vi "EAGLE Setup Screen V3.vi"(9 "TableIn":string[][](table)) -> (1 "TableOut":string[][](table), 2 "Exit":bool)   [LabVIEW 2015]
uses:
  Controls/Eagle Data.ctl
panel:
  in  "Down Button":bool
  in  "Up Button":bool
  in  "LimbusDistanceNumeric 2":dbl min=-1000.0 max=1000.0
  out "Eagle Data":T1
  in  "PulseEnergyNumeric":dbl=0.3 min=0.3 max=2.0 format="%#.2g"
  in  "LimbusDistanceNumeric":dbl min=-1000.0 max=1000.0
  in  "PulseIntervalNumeric":dbl=4.0 min=4.0 max=10.0
  in  "NumOfPulsesNumeric":u32=1 min=1 max=100
  in  "EyeColor":enum32{"Dark", "Bright"}(radio) caption="Eye Color"
  in  "EyeSelect":enum32{"Right Eye", "Left Eye"}(radio) caption="Eye"
  in  "TreatArea":enum32{"Upper 180", "Lower 180", "Full 360"}(radio) caption="Treatment Area"
  in  "ID":string caption="Patient ID"
  out "GUI Table":string[][](table)
  in  "Save":bool
  in  "PulseEnergySlide":dbl(slide)=1.0 caption="Average Pulse\nEnergy [mJ]" min=0.3 max=2.0 step=0.1 scale=0.3..2.0
  in  "LimbusDistanceSlider":dbl(slide)=1.0 caption="Distance From \nLimbus [um]" min=-1000.0 max=1000.0 step=0.1 scale=-1000.0..1000.0
  in  "PulseIntervalSlider":dbl(slide)=4.0 caption="Time Between \nPulses [mSec]" min=4.0 max=10.0 step=1.0 scale=4.0..10.0
  in  "NumOfPulsesSlider":u32(slide)=1 caption="Number of \nLaser Pulses" min=1 max=100 step=1 scale=1.0..100.0
  in  "FillSetupList":bool
  in  "Next":bool
  # "Treatment Settings"
  # "Eye Info"
  # "Laser Settings"
  # "Treatment Info"
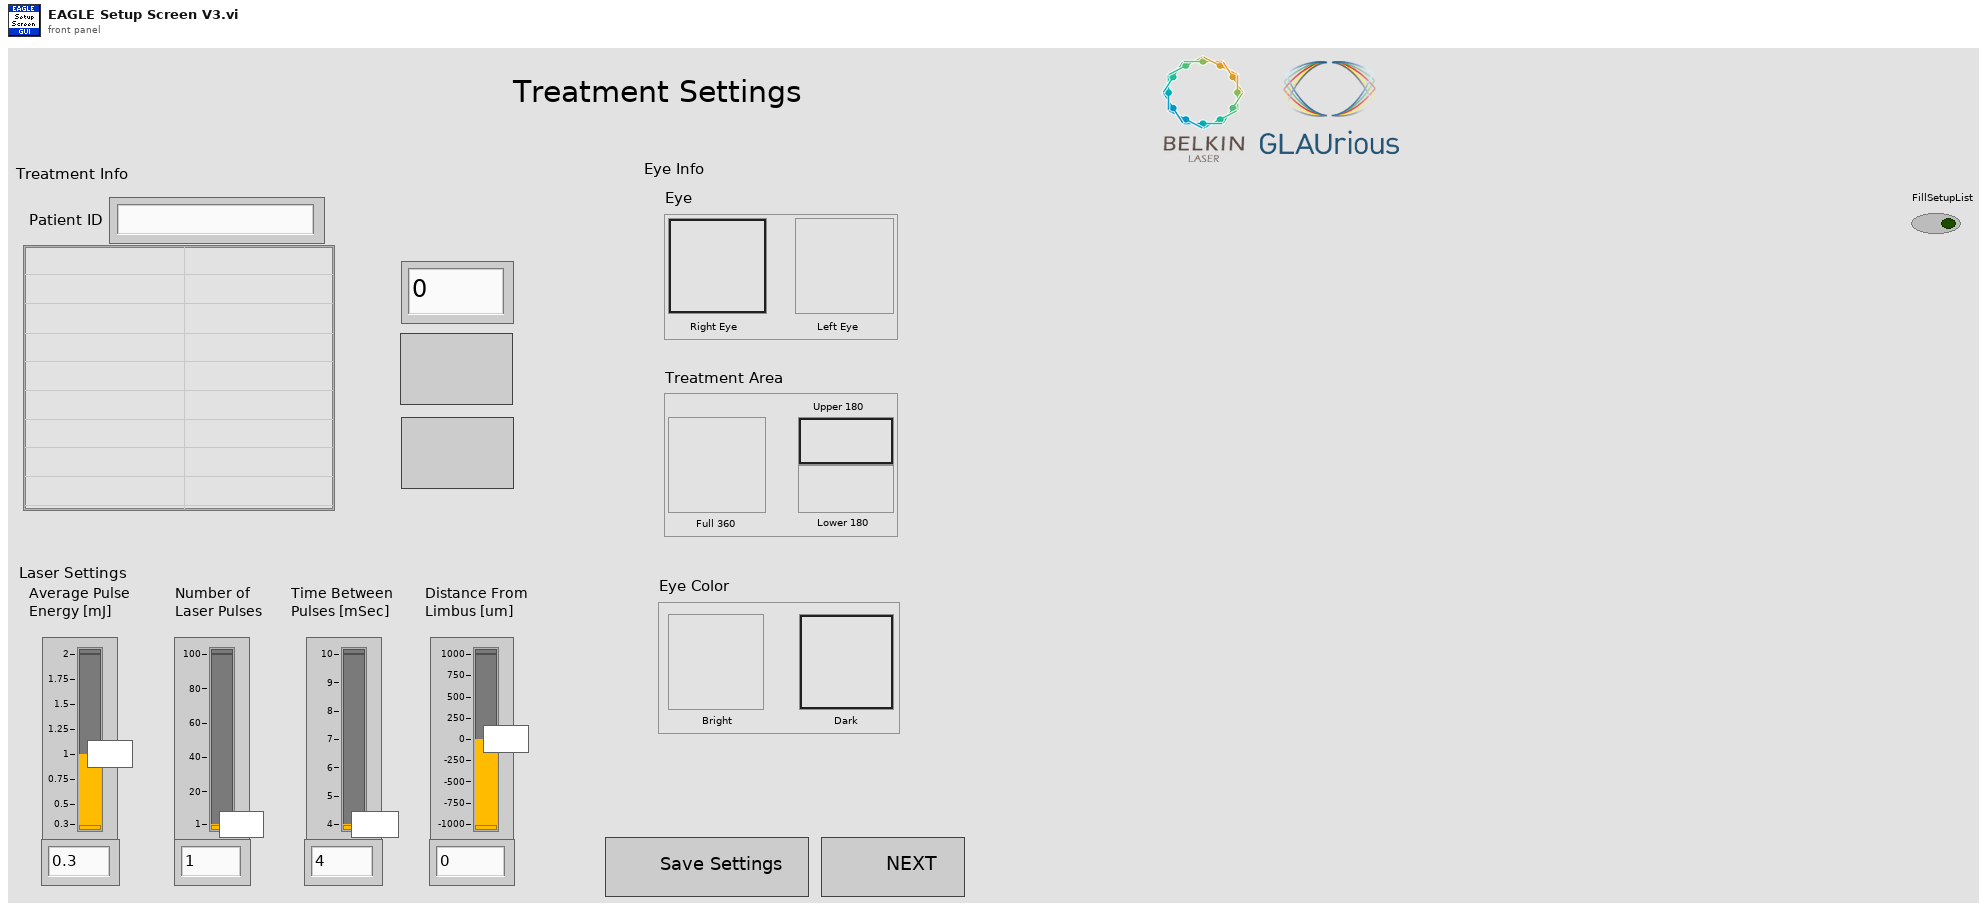
[diagram p1: front panel]
types:
  T1 = typedef "Eagle Data.ctl" = cluster{"Patient ID":string, "EyeSelect":enum32{"Right Eye", "Left Eye"}, "TreatArea":enum32{"Upper 180", "Lower 180", "Full 360"}, "EyeColor":enum32{"Dark", "Bright"}, "Laser Energy":dbl, "Number of pulses":u32, "Time between pulses":dbl, "Limbus distance":dbl, "Illumination Intensity":dbl, "Aiming Intensity":dbl, "Ranging Intensity":dbl}
  T2 = typedef "LVRectTypeDef.ctl" = cluster{"Left":i16, "Top":i16, "Right":i16, "Bottom":i16}
  T3 = typedef "LVPositionTypeDef.ctl" = cluster{"Left":i32, "Top":i32}
  T4 = cluster{"ID":string, "EyeSelect":enum32{"Right Eye", "Left Eye"}, "TreatArea":enum32{"Upper 180", "Lower 180", "Full 360"}, "EyeColor":enum32{"Dark", "Bright"}, "PulseEnergySlide":dbl, "NumOfPulsesSlider":u32, "PulseIntervalSlider":dbl, "LimbusDistanceSlider":dbl, "Illumination Intensity":dbl, "Aiming Intensity":dbl, "Ranging Intensity":dbl}
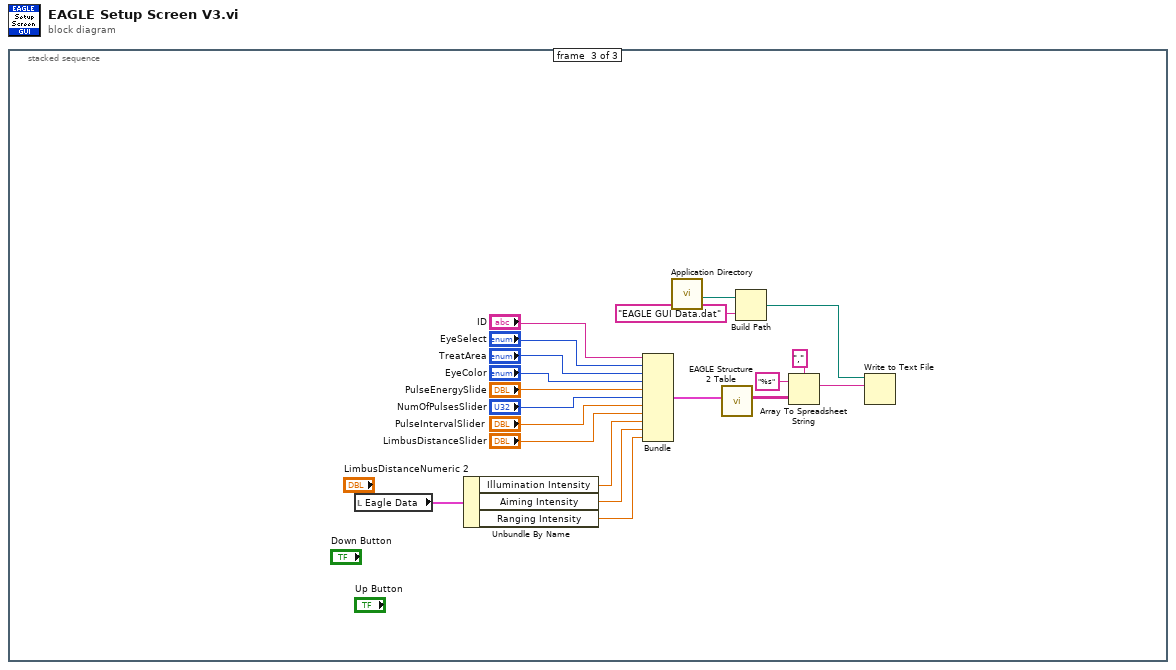
[diagram p0: block diagram]
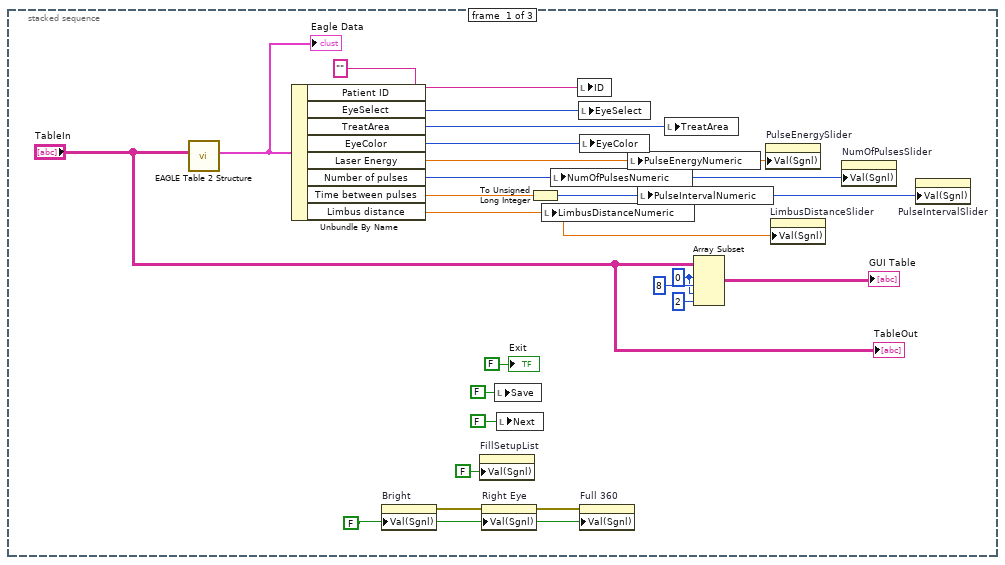
[diagram p2: hidden frame]
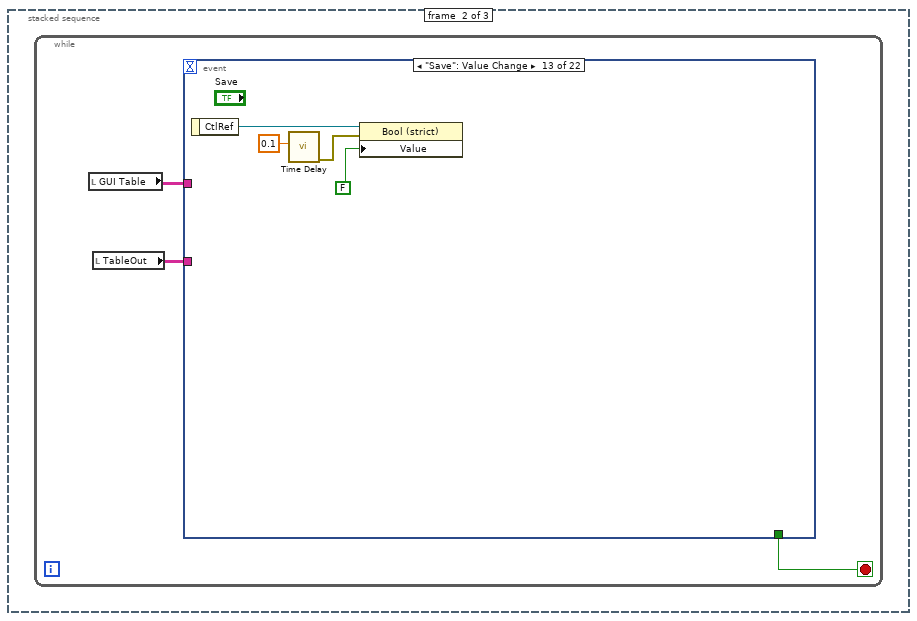
[diagram p3: hidden frame]
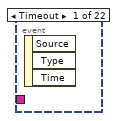
[diagram p4: hidden frame]
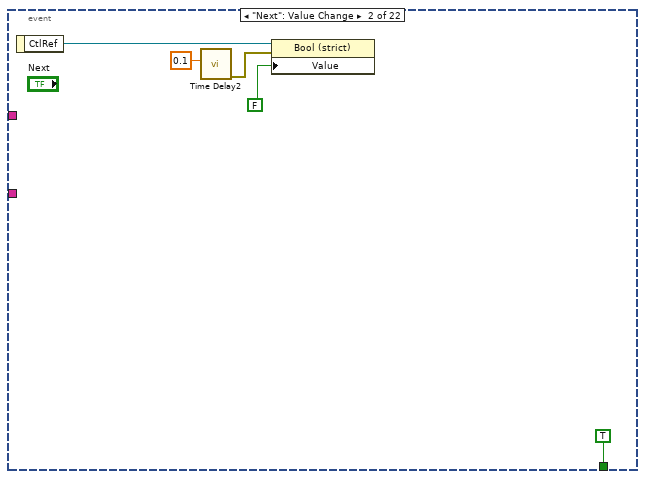
[diagram p5: hidden frame]
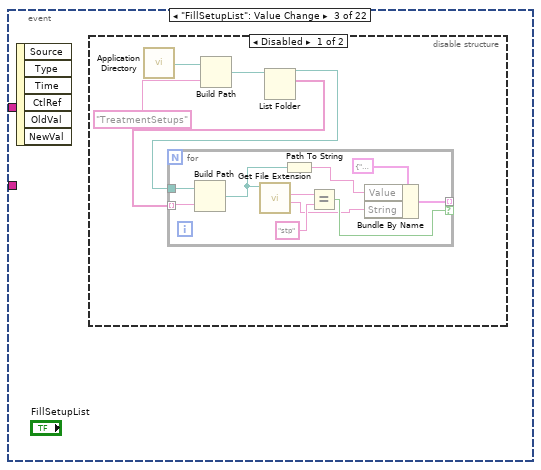
[diagram p6: hidden frame]
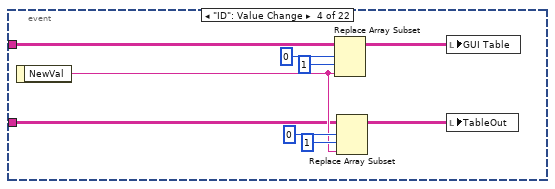
[diagram p8: hidden frame]
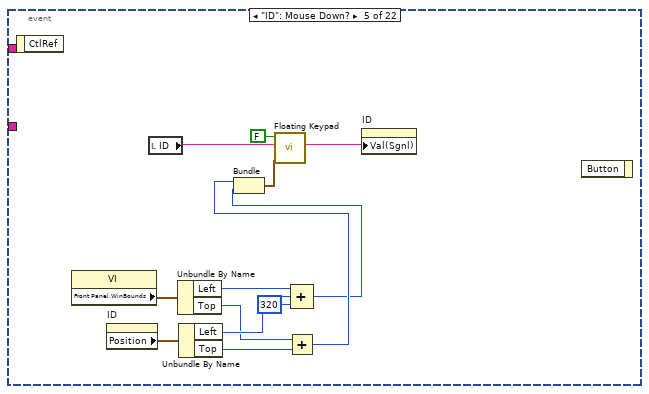
[diagram p9: hidden frame]
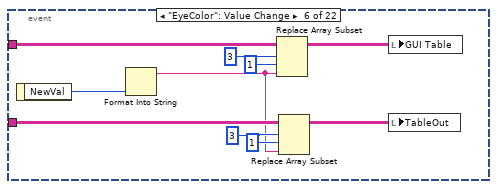
[diagram p10: hidden frame]
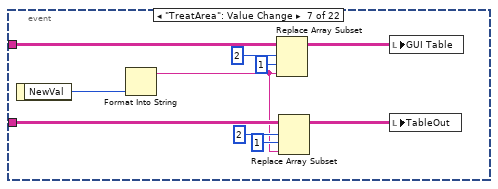
[diagram p11: hidden frame]
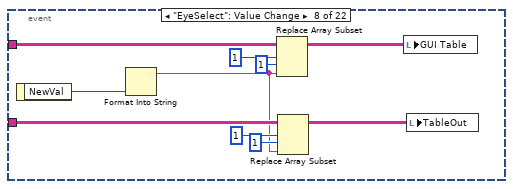
[diagram p12: hidden frame]
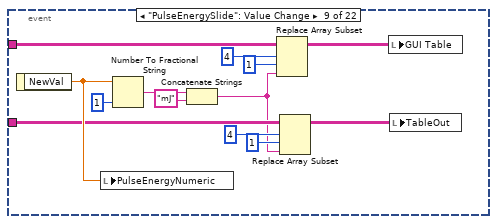
[diagram p13: hidden frame]
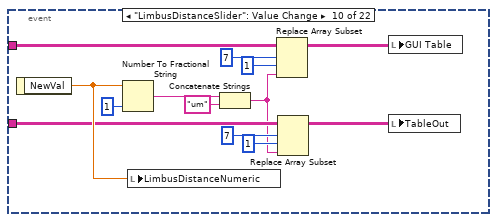
[diagram p14: hidden frame]
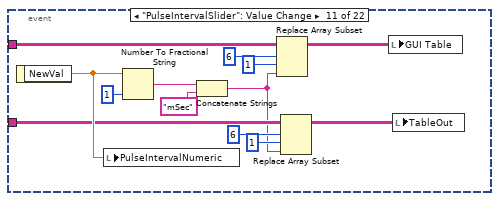
[diagram p15: hidden frame]
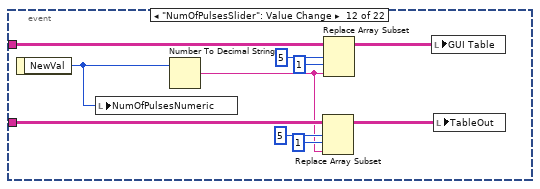
[diagram p16: hidden frame]
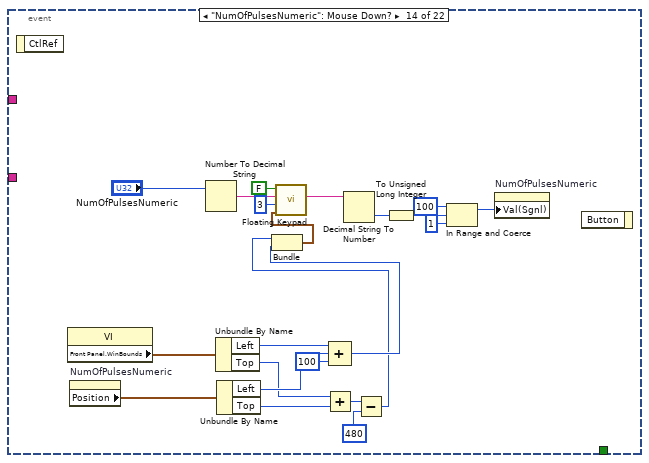
[diagram p17: hidden frame]
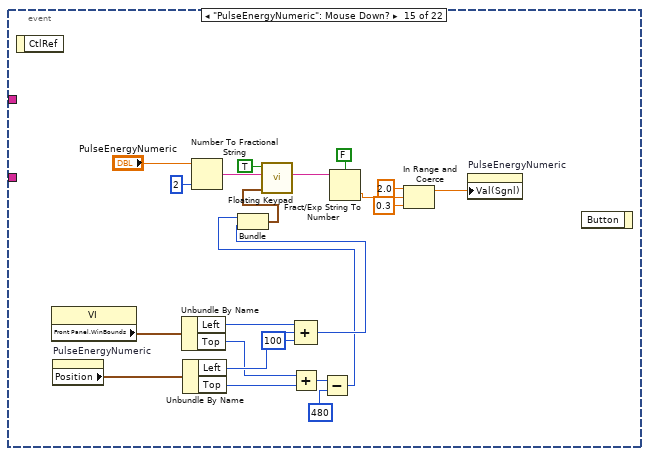
[diagram p18: hidden frame]
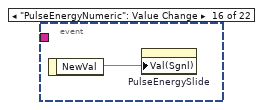
[diagram p19: hidden frame]
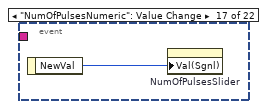
[diagram p20: hidden frame]
diagram:
  n1 = stacked-sequence {
    frame #0 {
      w5 = 0 ("index")
      w11 = FALSE
      n2 = call "EAGLE Table 2 Structure.vi"("Table Control"="TableIn") -> ("Eagle Data"=w7:T1)  [unwired: 10 in]
      "Eagle Data" <- w7
      n3 = Unbundle By Name(w7) -> ("EyeSelect"=w21:enum32{"Right Eye", "Left Eye"}, "TreatArea"=w20:enum32{"Upper 180", "Lower 180", "Full 360"}, "EyeColor"=w19:enum32{"Dark", "Bright"}, "Laser Energy"=w18:dbl, "Number of pulses"=w17:u32, "Time between pulses"=w16:dbl, "Limbus distance"=w14:dbl)  [unwired: 1 out]
      n4 = property on="Bright" class="Bool (strict)"("Val(Sgnl)"=w11) -> (error out=w9:errorcluster)  [unwired: 2 in, 1 out]
      n5 = property on="FillSetupList" class="Bool (strict)"("Val(Sgnl)"=FALSE ("Value (Signaling)")) -> ()  [unwired: 2 in, 2 out]
      n6 = property on="Right Eye" class="Bool (strict)"(error in=w9, "Val(Sgnl)"=w11) -> (error out=w10:errorcluster)  [unwired: 1 in, 1 out]
      n7 = local write "Save"(FALSE ("Save")) -> ()
      n8 = local write "Next"(FALSE ("Done")) -> ()
      n9 = To Unsigned Long Integer(number=w16) -> (unsigned 32bit integer=w15:u32)
      n10 = local write "LimbusDistanceNumeric"(w14) -> ()
      n11 = local write "NumOfPulsesNumeric"(w17) -> ()
      n12 = local write "ID"("" ("ID")) -> ()
      n13 = local write "EyeSelect"(w21) -> ()
      n14 = local write "EyeColor"(w19) -> ()
      n15 = property on="Full 360" class="Bool (strict)"(error in=w10, "Val(Sgnl)"=w11) -> ()  [unwired: 1 in, 2 out]
      n16 = local write "PulseEnergyNumeric"(w18) -> ()
      n17 = local write "PulseIntervalNumeric"(w15) -> ()
      n18 = local write "TreatArea"(w20) -> ()
      n19 = Array Subset(array="TableIn", index (row)=w5, length (row)=8 ("length"), index (col)=w5, length (col)=2 ("length")) -> (→"GUI Table":string[][])
      n20 = property on="PulseEnergySlider" class="Slide (strict)"("Val(Sgnl)"=w18) -> ()  [unwired: 2 in, 2 out]
      n21 = property on="LimbusDistanceSlider" class="Slide (strict)"("Val(Sgnl)"=w14) -> ()  [unwired: 2 in, 2 out]
      n22 = property on="NumOfPulsesSlider" class="Slide (strict)"("Val(Sgnl)"=w17) -> ()  [unwired: 2 in, 2 out]
      n23 = property on="PulseIntervalSlider" class="Slide (strict)"("Val(Sgnl)"=w15) -> ()  [unwired: 2 in, 2 out]
      "TableOut" <- "TableIn"
      "Exit" <- FALSE ("Exit")
    }
    frame #1 {
      n24 = while {
        stop <- w25 stop-if-true
        n25 = local read "GUI Table"() -> (w24:string[][])
        n26 = local read "TableOut"() -> (w23:string[][])
        n27 = event shown="[12] \"Save\": Value Change" {
          selector: _ -> [_ _ _ _ _ _ _ _ _ _ _ _ _ _ _ _ _ _ _ _ _ _]
          dyn-events: _ -> [_ _ _ _ _ _ _ _ _ _ _ _ _ _ _ _ _ _ _ _ _ _]
          timeout: _ -> [_ _ _ _ _ _ _ _ _ _ _ _ _ _ _ _ _ _ _ _ _ _]
          tunnel: [_ TRUE _ _ _ _ _ _ _ _ _ _ _ _ _ _ _ _ _ _ _ _] -> w25
          tunnel: w24 -> [_ _ _ w48 _ w68 w83 w93 w103 w116 w129 w142 _ _ _ _ _ _ _ _ _ _]
          tunnel: w23 -> [_ _ _ w47 _ w71 w80 w90 w100 w113 w126 w139 _ _ _ _ _ _ _ _ _ _]
          event Timeout {
            n28 = event-data() -> ()  [unwired: 1 in, 3 out]
          }
          event "Next": Value Change {
            n29 = event-data() -> ("CtlRef"=w26:refnum<vi>)  [unwired: 1 in]
            n30 = call "Time Delay2"("Delay Time (s)"=0.1) -> ("error out"=w28:errorcluster)  [unwired: 10 in]
            n31 = property class="Bool (strict)"(reference=w26, error in=w28, "Value"=FALSE) -> ()  [unwired: 2 out]
          }
          event "FillSetupList": Value Change {
            n32 = event-data() -> ()  [unwired: 1 in, 6 out]
            n33 = disable-structure shown="Disabled" {
              frame Disabled {
                n34 = call <vilib>:"Application Directory.vi"() -> ("Application Directory"=w35:path)
                n35 = Build Path(base path=w35, name or relative path="TreatmentSetups") -> (appended path=w33:path)
                n36 = List Folder(path=w33) -> (path out=w31:path, filenames=w32:string[])  [unwired: 3 in, 2 out]
                n37 = for {
                  tunnel: w32 -> [w40] mode=indexing
                  tunnel: w31 -> [w45]
                  tunnel: [w39] -> _ mode=indexing if=w38
                  n38 = Build Path(base path=w45, name or relative path=w40) -> (appended path=w43:path)
                  n39 = call <vilib>:"Get File Extension.vi"("file"=w43) -> ("filename without extension"=w36:string, "lowercase file extension"=w37:string)  [unwired: 6 in, 3 out]
                  n40 = Path To String(path=w43) -> (string=w41:string)
                  n41 = Equal?(x=w37, y="stp") -> (x = y?=w38:bool)
                  n42 = Bundle By Name(cluster=cluster{"String":string, "Value":string} {"String"="", "Value"=""}, "Value"=w41, "String"=w36) -> (w39:cluster{"String":string, "Value":string})
                }
              }
              frame Enabled {
              }
            }
          }
          event "ID": Value Change {
            n43 = event-data() -> ("NewVal"=w49:string)  [unwired: 1 in]
            n44 = Replace Array Subset(array=w48, new element=w49, index (row)=0 ("disabled index (row)"), index (col)=1 ("disabled index (col)")) -> (w54:string[][])
            n45 = Replace Array Subset(array=w47, new element=w49, index (row)=0 ("disabled index (row)"), index (col)=1 ("disabled index (col)")) -> (w46:string[][])
            n46 = local write "GUI Table"(w54) -> ()
            n47 = local write "TableOut"(w46) -> ()
          }
          event "ID": Mouse Down? {
            n48 = event-data() -> ()  [unwired: 1 in, 1 out]
            n49 = property class="VI"() -> ("Front Panel.WinBounds"=w64:T2)  [unwired: 2 in, 2 out]
            n50 = property on="ID" class="Str"() -> ("Position"=w63:T3)  [unwired: 2 in, 2 out]
            n51 = local read "ID"() -> (w67:string)
            n52 = Unbundle By Name(w64) -> ("Left"=w62:i16, "Top"=w59:i16)
            n53 = Unbundle By Name(w63) -> ("Left"=w61:i32, "Top"=w60:i32)
            n54 = Add(x=w59, y=w60) -> (x+y=w58:i32)
            n55 = Compound Arithmetic op=ADD(w62, w61, 320 ("value")) -> (w57:i32)
            n56 = Bundle(w58, w57) -> (w56:cluster{i32, i32})  [unwired: 1 in]
            n57 = call "Floating Keypad.vi"("Position"=w56, "StringIn"=w67, "Allow dot"=FALSE) -> ("StringOut"=w65:string)  [unwired: 8 in]
            n58 = property on="ID" class="Str"("Val(Sgnl)"=w65) -> ()  [unwired: 2 in, 2 out]
            n59 = event-data() -> ()  [unwired: 2 in, 1 out]
          }
          event "EyeColor": Value Change {
            n60 = event-data() -> ("NewVal"=w75:enum32{"Dark", "Bright"})  [unwired: 1 in]
            n61 = Format Into String(w75) -> (resulting string=w69:string)  [unwired: 3 in, 1 out]
            n62 = Replace Array Subset(array=w68, new element=w69, index (row)=3 ("disabled index (row)"), index (col)=1 ("disabled index (col)")) -> (w77:string[][])
            n63 = Replace Array Subset(array=w71, new element=w69, index (row)=3 ("disabled index (row)"), index (col)=1 ("disabled index (col)")) -> (w70:string[][])
            n64 = local write "GUI Table"(w77) -> ()
            n65 = local write "TableOut"(w70) -> ()
          }
          event "TreatArea": Value Change {
            n66 = event-data() -> ("NewVal"=w85:enum32{"Upper 180", "Lower 180", "Full 360"})  [unwired: 1 in]
            n67 = Format Into String(w85) -> (resulting string=w79:string)  [unwired: 3 in, 1 out]
            n68 = Replace Array Subset(array=w83, new element=w79, index (row)=2 ("disabled index (row)"), index (col)=1 ("disabled index (col)")) -> (w87:string[][])
            n69 = Replace Array Subset(array=w80, new element=w79, index (row)=2 ("disabled index (row)"), index (col)=1 ("disabled index (col)")) -> (w78:string[][])
            n70 = local write "GUI Table"(w87) -> ()
            n71 = local write "TableOut"(w78) -> ()
          }
          event "EyeSelect": Value Change {
            n72 = event-data() -> ("NewVal"=w95:enum32{"Right Eye", "Left Eye"})  [unwired: 1 in]
            n73 = Format Into String(w95) -> (resulting string=w89:string)  [unwired: 3 in, 1 out]
            n74 = Replace Array Subset(array=w93, new element=w89, index (row)=1 ("disabled index (row)"), index (col)=1 ("disabled index (col)")) -> (w97:string[][])
            n75 = Replace Array Subset(array=w90, new element=w89, index (row)=1 ("disabled index (row)"), index (col)=1 ("disabled index (col)")) -> (w88:string[][])
            n76 = local write "GUI Table"(w97) -> ()
            n77 = local write "TableOut"(w88) -> ()
          }
          event "PulseEnergySlide": Value Change {
            n78 = event-data() -> ("NewVal"=w104:dbl)  [unwired: 1 in]
            n79 = local write "PulseEnergyNumeric"(w104) -> ()
            n80 = Number To Fractional String(number=w104, precision (6)=i16 1) -> (F-format string=w105:string)  [unwired: 2 in]
            n81 = Concatenate Strings(w105, "mJ" ("string")) -> (w99:string)
            n82 = Replace Array Subset(array=w103, new element=w99, index (row)=4 ("disabled index (row)"), index (col)=1 ("disabled index (col)")) -> (w110:string[][])
            n83 = Replace Array Subset(array=w100, new element=w99, index (row)=4 ("disabled index (row)"), index (col)=1 ("disabled index (col)")) -> (w98:string[][])
            n84 = local write "GUI Table"(w110) -> ()
            n85 = local write "TableOut"(w98) -> ()
          }
          event "LimbusDistanceSlider": Value Change {
            n86 = event-data() -> ("NewVal"=w117:dbl)  [unwired: 1 in]
            n87 = Number To Fractional String(number=w117, precision (6)=i16 1) -> (F-format string=w118:string)  [unwired: 2 in]
            n88 = local write "LimbusDistanceNumeric"(w117) -> ()
            n89 = Concatenate Strings(w118, "um" ("string")) -> (w112:string)
            n90 = Replace Array Subset(array=w116, new element=w112, index (row)=7 ("disabled index (row)"), index (col)=1 ("disabled index (col)")) -> (w123:string[][])
            n91 = Replace Array Subset(array=w113, new element=w112, index (row)=7 ("disabled index (row)"), index (col)=1 ("disabled index (col)")) -> (w111:string[][])
            n92 = local write "GUI Table"(w123) -> ()
            n93 = local write "TableOut"(w111) -> ()
          }
          event "PulseIntervalSlider": Value Change {
            n94 = event-data() -> ("NewVal"=w130:dbl)  [unwired: 1 in]
            n95 = local write "PulseIntervalNumeric"(w130) -> ()
            n96 = Number To Fractional String(number=w130, precision (6)=i16 1) -> (F-format string=w131:string)  [unwired: 2 in]
            n97 = Concatenate Strings(w131, "mSec" ("string")) -> (w125:string)
            n98 = Replace Array Subset(array=w129, new element=w125, index (row)=6 ("disabled index (row)"), index (col)=1 ("disabled index (col)")) -> (w136:string[][])
            n99 = Replace Array Subset(array=w126, new element=w125, index (row)=6 ("disabled index (row)"), index (col)=1 ("disabled index (col)")) -> (w124:string[][])
            n100 = local write "GUI Table"(w136) -> ()
            n101 = local write "TableOut"(w124) -> ()
          }
          event "NumOfPulsesSlider": Value Change {
            n102 = event-data() -> ("NewVal"=w143:u32)  [unwired: 1 in]
            n103 = local write "NumOfPulsesNumeric"(w143) -> ()
            n104 = Number To Decimal String(number=w143) -> (decimal integer string=w138:string)  [unwired: 1 in]
            n105 = Replace Array Subset(array=w139, new element=w138, index (row)=5 ("disabled index (row)"), index (col)=1 ("disabled index (col)")) -> (w137:string[][])
            n106 = Replace Array Subset(array=w142, new element=w138, index (row)=5 ("disabled index (row)"), index (col)=1 ("disabled index (col)")) -> (w146:string[][])
            n107 = local write "GUI Table"(w146) -> ()
            n108 = local write "TableOut"(w137) -> ()
          }
          event "Save": Value Change {
            n109 = event-data() -> ("CtlRef"=w148:refnum<vi>)  [unwired: 1 in]
            n110 = call "Time Delay"("Delay Time (s)"=0.1) -> ("error out"=w149:errorcluster)  [unwired: 10 in]
            n111 = property class="Bool (strict)"(reference=w148, error in=w149, "Value"=FALSE) -> ()  [unwired: 2 out]
          }
          event "NumOfPulsesNumeric": Mouse Down? {
            n112 = event-data() -> ()  [unwired: 1 in, 1 out]
            n113 = property class="VI"() -> ("Front Panel.WinBounds"=w167:T2)  [unwired: 2 in, 2 out]
            n114 = property on="NumOfPulsesNumeric" class="DigNum (strict)"() -> ("Position"=w161:T3)  [unwired: 2 in, 2 out]
            n115 = Number To Decimal String(number="NumOfPulsesNumeric") -> (decimal integer string=w172:string)  [unwired: 1 in]
            n116 = Unbundle By Name(w167) -> ("Left"=w166:i16, "Top"=w163:i16)
            n117 = Unbundle By Name(w161) -> ("Left"=w165:i32, "Top"=w164:i32)
            n118 = Add(x=w163, y=w164) -> (x+y=w159:i32)
            n119 = Compound Arithmetic op=ADD(w166, w165, 100 ("value")) -> (w160:i32)
            n120 = Subtract(x=w159, y=480) -> (x-y=w157:i32)
            n121 = Bundle(w157, w160) -> (w156:cluster{i32, i32})  [unwired: 1 in]
            n122 = call "Floating Keypad.vi"("Position"=w156, "Length"=3, "StringIn"=w172, "Allow dot"=FALSE) -> ("StringOut"=w171:string)  [unwired: 7 in]
            n123 = Decimal String To Number(string=w171) -> (number=w170:i32)  [unwired: 2 in, 1 out]
            n124 = To Unsigned Long Integer(number=w170) -> (unsigned 32bit integer=w155:u32)
            n125 = In Range and Coerce(upper limit=u32 100, x=w155, lower limit=u32 1) -> (coerced(x)=w154:u32)  [unwired: 1 out]
            n126 = property on="NumOfPulsesNumeric" class="DigNum (strict)"("Val(Sgnl)"=w154) -> ()  [unwired: 2 in, 2 out]
            n127 = event-data() -> ()  [unwired: 2 in, 1 out]
          }
          event "PulseEnergyNumeric": Mouse Down? {
            n128 = event-data() -> ()  [unwired: 1 in, 1 out]
            n129 = property class="VI"() -> ("Front Panel.WinBounds"=w190:T2)  [unwired: 2 in, 2 out]
            n130 = property on="PulseEnergyNumeric" class="DigNum (strict)"() -> ("Position"=w179:T3)  [unwired: 2 in, 2 out]
            n131 = Unbundle By Name(w190) -> ("Left"=w189:i16, "Top"=w186:i16)
            n132 = Unbundle By Name(w179) -> ("Left"=w188:i32, "Top"=w187:i32)
            n133 = Number To Fractional String(number="PulseEnergyNumeric", precision (6)=i16 2) -> (F-format string=w194:string)  [unwired: 2 in]
            n134 = Add(x=w186, y=w187) -> (x+y=w183:i32)
            n135 = Compound Arithmetic op=ADD(w189, w188, 100 ("value")) -> (w184:i32)
            n136 = Subtract(x=w183, y=480) -> (x-y=w181:i32)
            n137 = Bundle(w181, w184) -> (w180:cluster{i32, i32})  [unwired: 1 in]
            n138 = call "Floating Keypad.vi"("Position"=w180, "StringIn"=w194, "Allow dot"=TRUE) -> ("StringOut"=w193:string)  [unwired: 8 in]
            n139 = Fract/Exp String To Number(use system decimal point (T)=FALSE, string=w193) -> (number=w176:dbl)  [unwired: 2 in, 1 out]
            n140 = In Range and Coerce(upper limit=2.0, x=w176, lower limit=0.3) -> (coerced(x)=w177:dbl)  [unwired: 1 out]
            n141 = property on="PulseEnergyNumeric" class="DigNum (strict)"("Val(Sgnl)"=w177) -> ()  [unwired: 2 in, 2 out]
            n142 = event-data() -> ()  [unwired: 2 in, 1 out]
          }
          event "PulseEnergyNumeric": Value Change {
            n143 = event-data() -> ("NewVal"=w195:dbl)  [unwired: 1 in]
            n144 = property on="PulseEnergySlide" class="Slide (strict)"("Val(Sgnl)"=w195) -> ()  [unwired: 2 in, 2 out]
          }
          event "NumOfPulsesNumeric": Value Change {
            n145 = event-data() -> ("NewVal"=w196:u32)  [unwired: 1 in]
            n146 = property on="NumOfPulsesSlider" class="Slide (strict)"("Val(Sgnl)"=w196) -> ()  [unwired: 2 in, 2 out]
          }
          event "PulseIntervalNumeric": Mouse Down? {
            n147 = event-data() -> ()  [unwired: 1 in, 1 out]
            n148 = property class="VI"() -> ("Front Panel.WinBounds"=w212:T2)  [unwired: 2 in, 2 out]
            n149 = property on="PulseIntervalNumeric" class="DigNum (strict)"() -> ("Position"=w201:T3)  [unwired: 2 in, 2 out]
            n150 = Unbundle By Name(w212) -> ("Left"=w211:i16, "Top"=w208:i16)
            n151 = Unbundle By Name(w201) -> ("Left"=w210:i32, "Top"=w209:i32)
            n152 = Number To Decimal String(number="PulseIntervalNumeric") -> (decimal integer string=w217:string)  [unwired: 1 in]
            n153 = Add(x=w208, y=w209) -> (x+y=w205:i32)
            n154 = Compound Arithmetic op=ADD(w211, w210, 100 ("value")) -> (w206:i32)
            n155 = Subtract(x=w205, y=480) -> (x-y=w203:i32)
            n156 = Bundle(w203, w206) -> (w202:cluster{i32, i32})  [unwired: 1 in]
            n157 = call "Floating Keypad.vi"("Position"=w202, "StringIn"=w217, "Allow dot"=FALSE) -> ("StringOut"=w216:string)  [unwired: 8 in]
            n158 = Decimal String To Number(string=w216) -> (number=w215:i32)  [unwired: 2 in, 1 out]
            n159 = To Unsigned Long Integer(number=w215) -> (unsigned 32bit integer=w200:u32)
            n160 = In Range and Coerce(upper limit=u32 10, x=w200, lower limit=u32 4) -> (coerced(x)=w199:u32)  [unwired: 1 out]
            n161 = property on="PulseIntervalNumeric" class="DigNum (strict)"("Val(Sgnl)"=w199) -> ()  [unwired: 2 in, 2 out]
            n162 = event-data() -> ()  [unwired: 2 in, 1 out]
          }
          event "PulseIntervalNumeric": Value Change {
            n163 = event-data() -> ("NewVal"=w218:dbl)  [unwired: 1 in]
            n164 = property on="PulseIntervalSlider" class="Slide (strict)"("Val(Sgnl)"=w218) -> ()  [unwired: 2 in, 2 out]
          }
          event "LimbusDistanceNumeric": Mouse Down? {
            n165 = event-data() -> ()  [unwired: 1 in, 1 out]
            n166 = property class="VI"() -> ("Front Panel.WinBounds"=w237:T2)  [unwired: 2 in, 2 out]
            n167 = property on="LimbusDistanceNumeric" class="DigNum (strict)"() -> ("Position"=w226:T3)  [unwired: 2 in, 2 out]
            n168 = Number To Fractional String(use system decimal point (T)=FALSE, number="LimbusDistanceNumeric", precision (6)=i16 1) -> (F-format string=w240:string)  [unwired: 1 in]
            n169 = Unbundle By Name(w237) -> ("Left"=w236:i16, "Top"=w233:i16)
            n170 = Unbundle By Name(w226) -> ("Left"=w235:i32, "Top"=w234:i32)
            n171 = Add(x=w233, y=w234) -> (x+y=w230:i32)
            n172 = Compound Arithmetic op=ADD(w236, w235, 100 ("value")) -> (w231:i32)
            n173 = Subtract(x=w230, y=480) -> (x-y=w228:i32)
            n174 = Bundle(w228, w231) -> (w227:cluster{i32, i32})  [unwired: 1 in]
            n175 = call "Floating Keypad.vi"("Position"=w227, "StringIn"=w240, "Allow dot"=TRUE) -> ("StringOut"=w239:string)  [unwired: 8 in]
            n176 = Fract/Exp String To Number(use system decimal point (T)=FALSE, string=w239) -> (number=w224:dbl)  [unwired: 2 in, 1 out]
            n177 = In Range and Coerce(upper limit=1000.0, x=w224, lower limit=-1000.0) -> (coerced(x)=w223:dbl)  [unwired: 1 out]
            n178 = property on="LimbusDistanceNumeric" class="DigNum (strict)"("Val(Sgnl)"=w223) -> ()  [unwired: 2 in, 2 out]
            n179 = event-data() -> ()  [unwired: 2 in, 1 out]
          }
          event "LimbusDistanceNumeric": Value Change {
            n180 = event-data() -> ("NewVal"=w242:dbl)  [unwired: 1 in]
            n181 = property on="LimbusDistanceSlider" class="Slide (strict)"("Val(Sgnl)"=w242) -> ()  [unwired: 2 in, 2 out]
          }
          event Panel Close? {
            n182 = event-data() -> ()  [unwired: 1 in, 1 out]
            n183 = Two Button Dialog(message="Press OK to quit the application") -> (T button?=w243:bool)  [unwired: 2 in]
            n184 = case shown="True" w243 {
              frame False {
              }
              frame True {
                n185 = property on="Next" class="Bool (strict)"("Val(Sgnl)"=FALSE ("Value (Signaling)")) -> ()  [unwired: 2 in, 2 out]
                n186 = local write "Exit"(TRUE ("Exit")) -> ()
              }
            }
            n187 = event-data("Discard?"=TRUE) -> ()  [unwired: 1 in, 1 out]
          }
        }
      }
    }
    frame #2 {
      n188 = local read "Eagle Data"() -> (w260:T1)
      n189 = Unbundle By Name(w260) -> ("Illumination Intensity"=w259:dbl, "Aiming Intensity"=w258:dbl, "Ranging Intensity"=w257:dbl)
      n190 = Bundle("ID"="ID", "EyeSelect"="EyeSelect", "TreatArea"="TreatArea", "EyeColor"="EyeColor", "PulseEnergySlide"="PulseEnergySlide", "NumOfPulsesSlider"="NumOfPulsesSlider", "PulseIntervalSlider"="PulseIntervalSlider", "LimbusDistanceSlider"="LimbusDistanceSlider", "Illumination Intensity"=w259, "Aiming Intensity"=w258, "Ranging Intensity"=w257) -> (w261:T4)  [unwired: 1 in]
      n191 = call <vilib>:"Application Directory.vi"() -> ("Application Directory"=w250:path)
      n192 = call "EAGLE Structure 2 Table.vi"("Eagle Data"=w261) -> ("TableOut"=w254:string[][])  [unwired: 10 in]
      n193 = Build Path(base path=w250, name or relative path="EAGLE GUI Data.dat") -> (appended path=w248:path)
      n194 = Array To Spreadsheet String(delimiter (Tab)=",", array=w254, 3:"%s" ("format string")) -> (spreadsheet string=w251:string)
      n195 = Write to Text File(file (use dialog)=w248, text=w251) -> ()  [unwired: 2 in, 3 out]
    }
  }
